vi "Convert Header Text to Image.vi"(8 "Enum":enum16{"LEFT", "CENTER", "RIGHT"}(ring), 9 "image path":string, 10 "text above image":string, 11 "HTML In":string) -> (3 "HTML Out":string)   [LabVIEW 2017, in "NI_ReportGenerationCore.lvlib"]
uses:
  <vilib>/Utility/NIReport.llb/NI_ReportGenerationCore.lvlib
  <vilib>/Utility/NIReport.llb/HTML Report Image Alignment.ctl
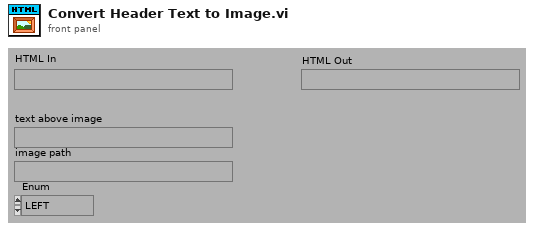
[diagram p1: front panel]
types:
  T1 = typedef "NI_ReportGenerationCore.lvlib/HTML Report Image Alignment.ctl" = enum16{"(default)", "LEFT", "RIGHT", "TOP", "TEXTTOP", "MIDDLE", "ABSMIDDLE", "BASELINE", "BOTTOM", "ABSBOTTOM"}
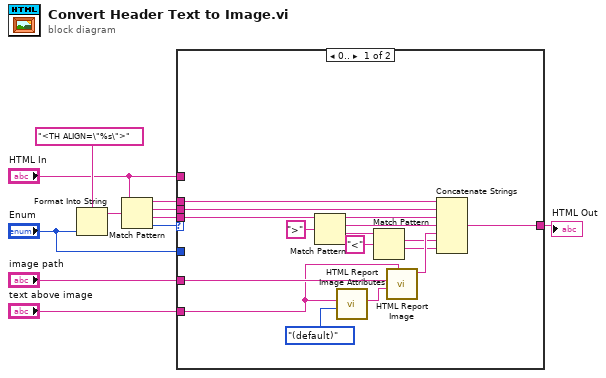
[diagram p0: block diagram]
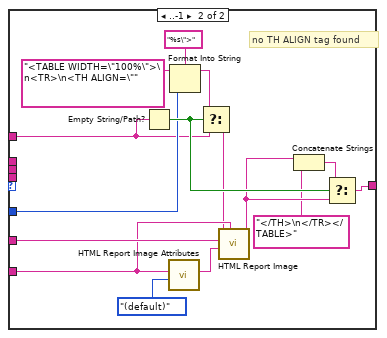
[diagram p2: hidden frame]
diagram:
  n1 = Format Into String(format string="<TH ALIGN=\"%s\">" ("Format String"), "Enum") -> (resulting string=w8:string)  [unwired: 2 in, 1 out]
  n2 = Match Pattern(string="HTML In", regular expression=w8) -> (before substring=w6:string, match substring=w5:string, after substring=w7:string, offset past match=w1:i32)  [unwired: 1 out]
  n3 = case shown="0.." w1 {
    tunnel: "image path" -> [w27 w42]
    tunnel: "text above image" -> [w26 w41]
    tunnel: w7 -> [w22 _]
    tunnel: w6 -> [w17 _]
    tunnel: w5 -> [w16 _]
    tunnel: [w15 w36] -> w4
    tunnel: "HTML In" -> [_ w30]
    tunnel: "Enum" -> [_ w32]
    frame 0.. {
      n4 = Match Pattern(string=w22, regular expression=">") -> (before substring=w21:string, match substring=w20:string, after substring=w19:string)  [unwired: 2 out]
      n5 = call <vilib>:"HTML Report Image Attributes.vi"("alignment (default)"=HTML_Report_Image_Alignment."(default)", "alt - alternative string"=w26) -> ("attributes out"=w25:string)  [unwired: 5 out]
      n6 = Match Pattern(string=w19, regular expression="<") -> (match substring=w13:string, after substring=w12:string)  [unwired: 3 out]
      n7 = call <vilib>:"HTML Report Image.vi"("label"=w26, "image attributes"=w25, "src - URL of image to embed"=w27) -> ("HTML out"=w14:string)  [unwired: 1 in, 7 out]
      n8 = Concatenate Strings(w17, w16, w21, w20, w14, w13, w12) -> (w15:string)
    }
    frame ..-1 {
      # "no TH ALIGN tag found"
      n9 = Empty String/Path?(string/path=w30) -> (empty?=w38:bool)
      n10 = call <vilib>:"HTML Report Image Attributes.vi"("alignment (default)"=HTML_Report_Image_Alignment."(default)", "alt - alternative string"=w41) -> ("attributes out"=w40:string)  [unwired: 5 out]
      n11 = Format Into String(format string="%s\">" ("Format String"), initial string="<TABLE WIDTH=\"100%\">\n<TR>\n<TH ALIGN=\"" ("Input String"), w32) -> (resulting string=w31:string)  [unwired: 1 in, 1 out]
      n12 = Select(t=w31, s=w38, f=w30) -> (s? t:f=w29:string)
      n13 = call <vilib>:"HTML Report Image.vi"("label"=w41, "image attributes"=w40, "src - URL of image to embed"=w42, "HTML in"=w29) -> ("HTML out"=w35:string)  [unwired: 7 out]
      n14 = Concatenate Strings(w35, "</TH>\n</TR></TABLE>" ("Substring")) -> (w37:string)
      n15 = Select(t=w37, s=w38, f=w35) -> (s? t:f=w36:string)
    }
  }
  "HTML Out" <- w4
